vi "5.vi"() -> ()   [LabVIEW 2015]
panel:
  out "Waveform Chart":dbl[](graph)
  out "Array":dbl[](array[numeric])
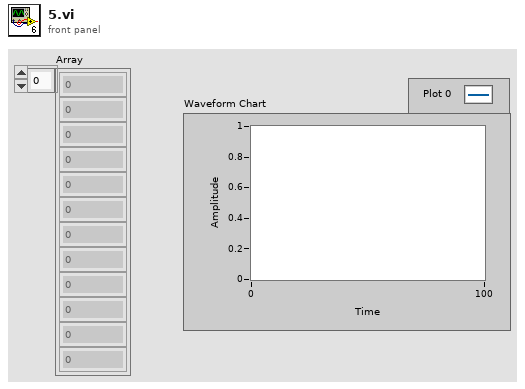
[diagram p1: front panel]
types:
  T1 = enum16{"open", "replace", "create", "open or create", "replace or create", "replace or create with confirmation"}
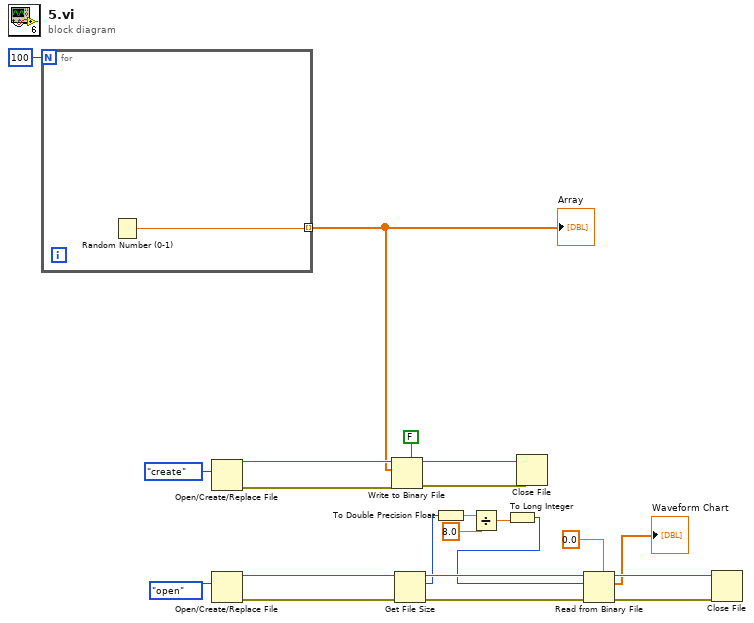
[diagram p0: block diagram]
diagram:
  n1 = for {
    N: 100 -> [_]
    tunnel: [w23] -> w16 mode=indexing
    n2 = Random Number (0-1)() -> (number: 0 to 1=w23:dbl)
  }
  "Array" <- w16
  n3 = Open/Create/Replace File(operation (0:open)=T1."create") -> (refnum out=w18:refnum<file>, error out=w19:errorcluster)  [unwired: 5 in, 1 out]
  n4 = Open/Create/Replace File(operation (0:open)=T1."open") -> (refnum out=w12:refnum<file>, error out=w13:errorcluster)  [unwired: 5 in, 1 out]
  n5 = Write to Binary File(file (use dialog)=w18, data=w16, error in=w19, 5:FALSE ("prepend array or string size? (T)")) -> (refnum out=w20:refnum<file>, error out=w21:errorcluster)  [unwired: 2 in, 1 out]
  n6 = Get File Size(file=w12, error in=w13) -> (refnum out=w11:refnum<file>, size (in bytes)=w5:i64, 0:w8:errorcluster)
  n7 = To Double Precision Float(number=w5) -> (double precision float=w7:dbl)
  n8 = Divide(x=w7, y=8.0) -> (x/y=w4:dbl)
  n9 = To Long Integer(number=w4) -> (32bit integer=w3:i32)
  n10 = Close File(refnum=w20, error in=w21) -> ()  [unwired: 2 out]
  n11 = Read from Binary File(5:0.0, 8:w8, 10:w3, 11:w11) -> (0:w10:errorcluster, 2:→"Waveform Chart":dbl[], 3:w9:refnum<file>)  [unwired: 2 in, 1 out]
  n12 = Close File(refnum=w9, error in=w10) -> ()  [unwired: 2 out]
